vi "Update File Name.vi"(8 "error in":errorcluster, 11 "Report Viewer in":refnum<class "Report Viewer.lvclass">) -> (0 "error out":errorcluster, 3 "Report Viewer out":refnum<class "Report Viewer.lvclass">)   [LabVIEW 2023, in "Report Viewer.lvlib" / "Report Viewer.lvclass"]
uses:
  Library/Report Viewer.lvclass
  Library/Report Viewer.lvclass/Report Viewer.ctl
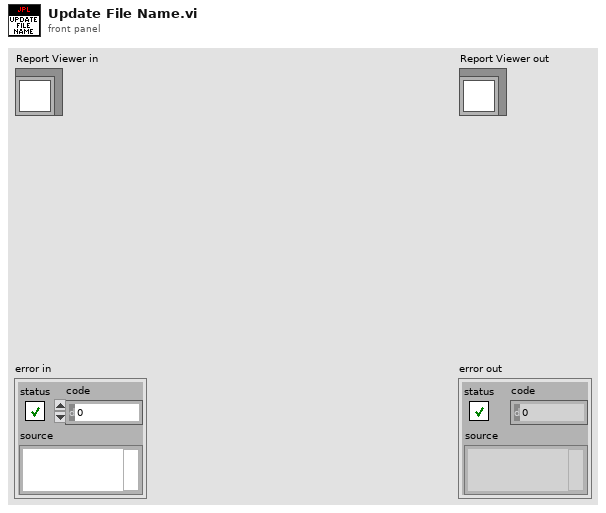
[diagram p1: front panel]
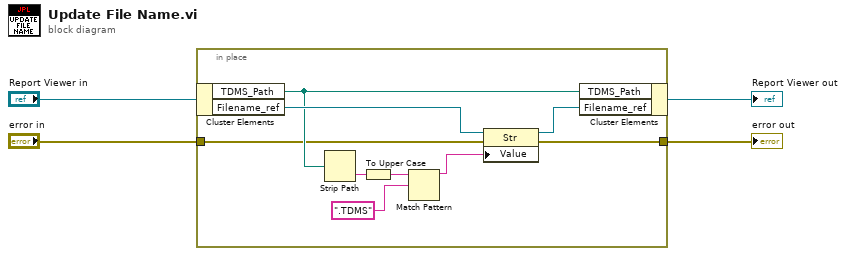
[diagram p0: block diagram]
diagram:
  n1 = in-place {
    in-place-border: "error in" -> [w6]
    in-place-border: [w5] -> w1
    n2 = in-place-cluster #1("Report Viewer in") -> ("TDMS_Path"=w11:path, "Filename_ref"=w13:refnum<vi>)
    n3 = Strip Path(path=w11) -> (name=w10:string)  [unwired: 1 out]
    n4 = To Upper Case(1:w10) -> (0:w7:string)
    n5 = Match Pattern(string=w7, regular expression=".TDMS") -> (before substring=w9:string)  [unwired: 1 in, 3 out]
    n6 = property class="Str"(reference=w13, error in=w6, "Value"=w9) -> (reference out=w12:refnum<vi>, error out=w5:errorcluster)
    n7 = in-place-cluster #1("TDMS_Path"=w11, "Filename_ref"=w12) -> (→"Report Viewer out":refnum<class "Report Viewer.lvclass">)
  }
  "error out" <- w1
